vi "Drive Station HUD.vi"() -> ()   [LabVIEW 2018]
uses:
  <vilib>/Rock Robotics/Network Tables/NT Read Number.vi
  <vilib>/Rock Robotics/Network Tables/NT Read Boolean.vi
  <vilib>/vision/NI_Vision_Development_Module.lvlib
panel:
  out "Final Image":T1(plugin-control)
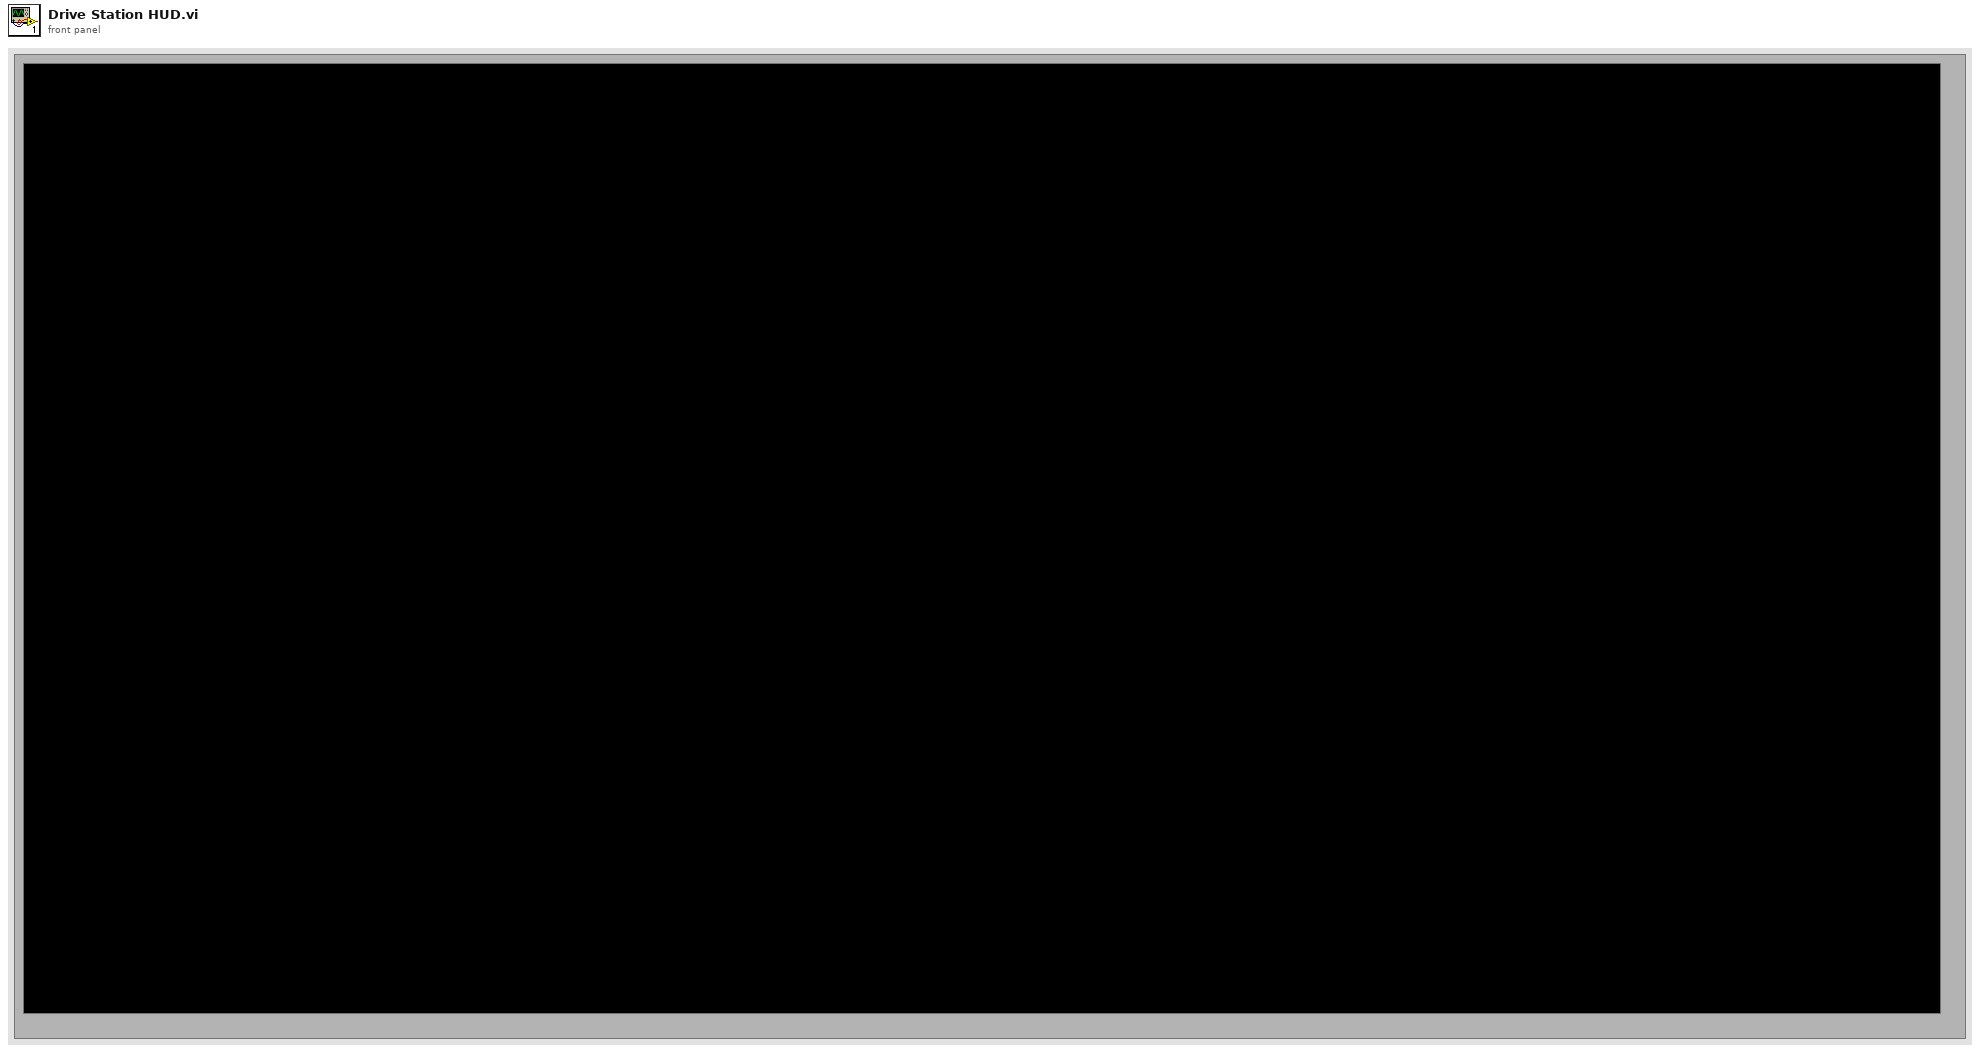
[diagram p1: front panel]
types:
  T1 = typedef "IMAQ Image.ctl" = refnum<image>
  T2 = enum32{"Invalid", "Standard", "Closed", "Hidden", "Minimized", "Maximized"}
  T3 = typedef "LVAllMonitorsDisplayTypeDef.ctl" = cluster{"Bounds":cluster{"Left":i16, "Top":i16, "Right":i16, "Bottom":i16}, "Depth":i16}[]
  T4 = cluster{"Left":i16, "Top":i16, "Right":i16, "Bottom":i16}
  T5 = cluster{"Left":i32, "Top":i32, "Right":i32, "Bottom":i32}
  T6 = cluster{"Desired Font (Application)":enum16{"User-specified Font", "Application Font", "System Font", "Dialog Font"}, "[User-specified Font]":cluster{"Font Name":string, "Size":i16, "Strikeout?":bool, "Italic?":bool, "Underline?":bool, "Outline?":bool, "Shadow?":bool, "Bold?":bool, "Rotation Angle":dbl}, "Horizontal Alignment":i16, "Vertical Alignment":i16}
  T7 = typedef "Image Type" = u32
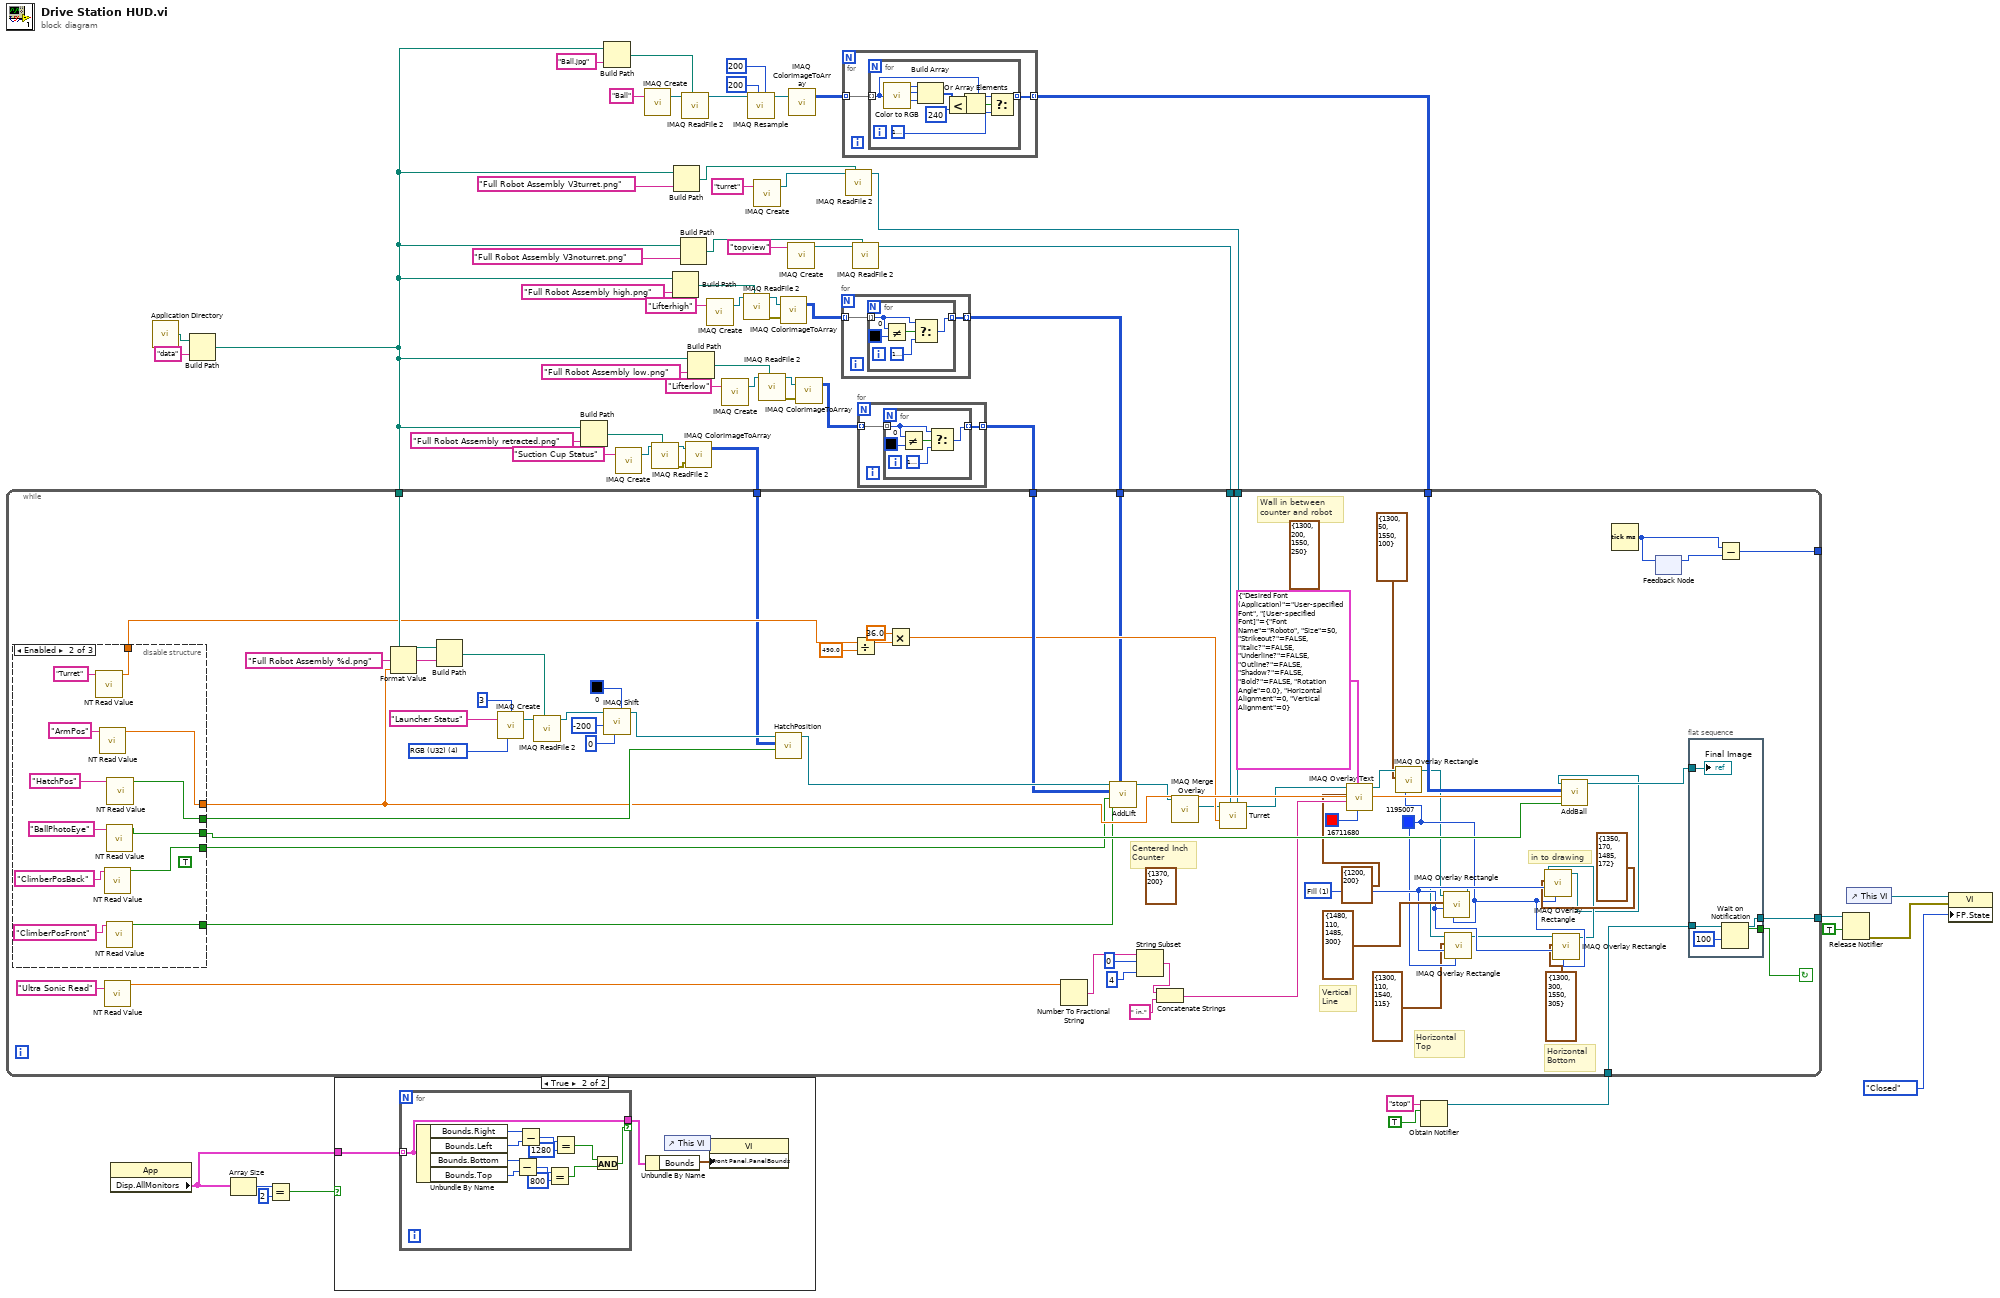
[diagram p0: block diagram]
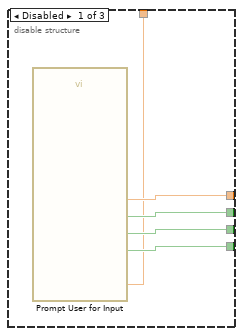
[diagram p2: hidden frame]
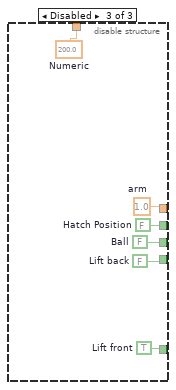
[diagram p3: hidden frame]
diagram:
  n1 = property class="App"() -> ("Disp.AllMonitors"=w55:T3)  [unwired: 2 in, 2 out]
  n2 = call <vilib>:"Application Directory.vi"() -> ("Application Directory"=w53:path)
  n3 = Build Path(base path=w53, name or relative path="data") -> (appended path=w1:path)
  n4 = Array Size(array=w55) -> (size(s)=w58:i32)
  n5 = Equal?(x=w58, y=2) -> (x = y?=w56:bool)
  n6 = case shown="True" w56 {
    tunnel: w55 -> [_ w62]
    frame False {
    }
    frame True {
      n7 = for {
        tunnel: w62 -> [w64] mode=indexing
        tunnel: [w64] -> w60 if=w63
        n8 = Unbundle By Name(w64) -> ("Bounds.Right"=w74:i16, "Bounds.Left"=w73:i16, "Bounds.Bottom"=w72:i16, "Bounds.Top"=w71:i16)
        n9 = Subtract(x=w72, y=w71) -> (x-y=w70:i16)
        n10 = Subtract(x=w74, y=w73) -> (x-y=w67:i16)
        n11 = Equal?(x=w70, y=i16 800) -> (x = y?=w65:bool)
        n12 = Equal?(x=w67, y=i16 1280) -> (x = y?=w66:bool)
        n13 = And(x=w66, y=w65) -> (x .and. y?=w63:bool)
      }
      n14 = Unbundle By Name(w60) -> ("Bounds"=w59:T4)
      n15 = control-ref of="This VI"() -> (w61:refnum<vi>)
      n16 = property class="VI"(reference=w61, "Front Panel.PanelBounds"=w59) -> ()  [unwired: 1 in, 2 out]
    }
  }
  n17 = Build Path(base path=w1, name or relative path="Full Robot Assembly retracted.png") -> (appended path=w14:path)
  n18 = Build Path(base path=w1, name or relative path="Ball.jpg") -> (appended path=w52:path)
  n19 = call "IMAQ Create"("Image Name"="Suction Cup Status") -> ("New Image"=w11:T1)  [unwired: 4 in, 1 out]
  n20 = call "IMAQ Create"("Image Name"="Ball") -> ("New Image"=w48:T1)  [unwired: 4 in, 1 out]
  n21 = call "IMAQ ReadFile 2"("File Path"=w14, "Image"=w11) -> ("error out"=w13:errorcluster, "Image Out"=w16:T1)  [unwired: 5 in, 3 out]
  n22 = Build Path(base path=w1, name or relative path="Full Robot Assembly high.png") -> (appended path=w2:path)
  n23 = Build Path(base path=w1, name or relative path="Full Robot Assembly V3turret.png") -> (appended path=w19:path)
  n24 = Build Path(base path=w1, name or relative path="Full Robot Assembly V3noturret.png") -> (appended path=w26:path)
  n25 = call "IMAQ ReadFile 2"("File Path"=w52, "Image"=w48) -> ("Image Out"=w49:T1)  [unwired: 5 in, 4 out]
  n26 = call "IMAQ ColorImageToArray"("Image"=w16, "error in (no error)"=w13) -> ("Image Pixels (U32)"=w10:u32[][])  [unwired: 2 in, 2 out]
  n27 = Build Path(base path=w1, name or relative path="Full Robot Assembly low.png") -> (appended path=w41:path)
  n28 = call "IMAQ Create"("Image Name"="Lifterhigh") -> ("New Image"=w5:T1)  [unwired: 4 in, 1 out]
  n29 = call "IMAQ Create"("Image Name"="Lifterlow") -> ("New Image"=w38:T1)  [unwired: 4 in, 1 out]
  n30 = call "IMAQ ReadFile 2"("File Path"=w2, "Image"=w5) -> ("error out"=w3:errorcluster, "Image Out"=w4:T1)  [unwired: 5 in, 3 out]
  n31 = call "IMAQ Resample"("X Resolution"=200, "Y Resolution"=200 ("X Resolution"), "Image Src"=w49) -> ("Image Dst Out"=w50:T1)  [unwired: 7 in, 1 out]
  n32 = call "IMAQ Create"("Image Name"="turret") -> ("New Image"=w20:T1)  [unwired: 4 in, 1 out]
  n33 = call "IMAQ ReadFile 2"("File Path"=w41, "Image"=w38) -> ("error out"=w40:errorcluster, "Image Out"=w39:T1)  [unwired: 5 in, 3 out]
  n34 = call "IMAQ ColorImageToArray"("Image"=w4, "error in (no error)"=w3) -> ("Image Pixels (U32)"=w9:u32[][])  [unwired: 2 in, 2 out]
  n35 = call "IMAQ Create"("Image Name"="topview") -> ("New Image"=w25:T1)  [unwired: 4 in, 1 out]
  n36 = call "IMAQ ColorImageToArray"("Image"=w50) -> ("Image Pixels (U32)"=w51:u32[][])  [unwired: 3 in, 2 out]
  n37 = call "IMAQ ColorImageToArray"("Image"=w39, "error in (no error)"=w40) -> ("Image Pixels (U32)"=w42:u32[][])  [unwired: 2 in, 2 out]
  n38 = for {
    tunnel: w9 -> [w76] mode=indexing
    tunnel: [w75] -> w8 mode=indexing
    n39 = for {
      tunnel: w76 -> [w79] mode=indexing
      tunnel: [w78] -> w75 mode=indexing
      n40 = Not Equal?(x=w79, y=u32 0) -> (x != y?=w80:bool)
      n41 = Select(t=w79, s=w80, f=u32 16777216) -> (s? t:f=w78:u32)
    }
  }
  n42 = for {
    tunnel: w51 -> [w83] mode=indexing
    tunnel: [w82] -> w43 mode=indexing
    n43 = for {
      tunnel: w83 -> [w85] mode=indexing
      tunnel: [w93] -> w82 mode=indexing
      n44 = call <vilib>:"Color to RGB.vi"("Color"=w85) -> ("Resolved Color"=w91:u32, "R"=w90:u8, "G"=w89:u8)  [unwired: 1 out]
      n45 = Build Array(w91, w90, w89) -> (w87:u32[])
      n46 = Less?(x=w87, y=240) -> (x < y?=w88:bool[])
      n47 = Or Array Elements(Boolean array=w88) -> (logical OR=w84:bool)
      n48 = Select(t=w85, s=w84, f=u32 16777216) -> (s? t:f=w93:u32)
    }
  }
  n49 = call "IMAQ ReadFile 2"("File Path"=w19, "Image"=w20) -> ("Image Out"=w17:T1)  [unwired: 5 in, 4 out]
  n50 = call "IMAQ ReadFile 2"("File Path"=w26, "Image"=w25) -> ("Image Out"=w22:T1)  [unwired: 5 in, 4 out]
  n51 = for {
    tunnel: w42 -> [w95] mode=indexing
    tunnel: [w94] -> w35 mode=indexing
    n52 = for {
      tunnel: w95 -> [w98] mode=indexing
      tunnel: [w97] -> w94 mode=indexing
      n53 = Not Equal?(x=w98, y=u32 0) -> (x != y?=w99:bool)
      n54 = Select(t=w98, s=w99, f=u32 16777216) -> (s? t:f=w97:u32)
    }
  }
  n55 = Obtain Notifier(name (unnamed)="stop", notification data type=TRUE) -> (notifier out=w32:refnum<notifier>)  [unwired: 2 in, 2 out]
  n56 = while {
    tunnel: w1 -> [w156]
    tunnel: w43 -> [w155]
    tunnel: w35 -> [w154]
    tunnel: w32 -> [w150]
    tunnel: [w149] -> w31
    tunnel: w22 -> [w134]
    tunnel: w17 -> [w132]
    tunnel: w10 -> [w130]
    tunnel: w8 -> [w129]
    tunnel: [w126] -> _
    stop <- w143 continue-if-true
    w110 = u32 1 items=["Frame", "Fill", "Highlight"] ("Drawing Mode (Frame)")
    (unwired) T5 {"Left"=1300, "Top"=200, "Right"=1550, "Bottom"=250} ("Rectangle")
    w107 = u32 1195007 ("Color")
    (unwired) cluster{"X":i32, "Y":i32} {"X"=1370, "Y"=200} ("Origin")
    w163 = T7 4 items=["Grayscale (U8)", "Grayscale (I16)", "Grayscale (SGL)", "Complex (CSG)", "RGB (U32)", "HSL (U32)", "RGB (U64)", "Grayscale (U16)"] ("Image Type")
    # "Horizontal\nBottom"
    # "Horizontal\nTop"
    # "Vertical\nLine"
    # "in to drawing"
    # "Centered Inch\nCounter"
    # "Wall in between \ncounter and robot"
    n57 = disable-structure shown="Enabled" {
      disable-tunnel: [w175 w183 w193] -> w153
      disable-tunnel: [w174 w184 w192] -> w152
      disable-tunnel: [w173 w186 w189] -> w151
      disable-tunnel: [w172 w185 w191] -> w142
      disable-tunnel: [w170 w177 w188] -> w148
      disable-tunnel: [_ w176 w190] -> w136
      frame Disabled {
        n58 = call "Prompt User for Input"() -> ("turret angle"=w170:dbl, "Invert Colors"=w171:bool, "Lifter extended"=w172:bool, "Ball Obtained"=w174:bool, "Suction Cup extended"=w175:bool, "Position of Launcher:"=w173:dbl)  [unwired: 12 in, 2 out]
      }
      frame Enabled {
        (unwired) TRUE ("Invert Colors")
        n59 = call-poly <vilib>:"NT Read Value.vi"("Name"="Turret") -> ("Numeric"=w177:dbl)  [unwired: 9 in, 1 out]
        n60 = call-poly <vilib>:"NT Read Value.vi"("Name"="ArmPos") -> ("Numeric"=w186:dbl)  [unwired: 9 in, 1 out]
        n61 = call-poly <vilib>:"NT Read Value.vi"("Name"="ClimberPosBack") -> ("Boolean"=w185:bool)  [unwired: 9 in, 1 out]
        n62 = call-poly <vilib>:"NT Read Value.vi"("Name"="BallPhotoEye") -> ("Boolean"=w184:bool)  [unwired: 9 in, 1 out]
        n63 = call-poly <vilib>:"NT Read Value.vi"("Name"="ClimberPosFront") -> ("Boolean"=w176:bool)  [unwired: 9 in, 1 out]
        n64 = call-poly <vilib>:"NT Read Value.vi"("Name"="HatchPos") -> ("Boolean"=w183:bool)  [unwired: 9 in, 1 out]
      }
      frame Disabled {
        w188 = 200.0  # Numeric
        w189 = 1.0  # arm
        w190 = TRUE  # Lift front
        w191 = FALSE  # Lift back
        w192 = FALSE  # Ball
        w193 = FALSE  # Hatch Position
      }
    }
    n65 = call-poly <vilib>:"NT Read Value.vi"("Name"="Ultra Sonic Read") -> ("Numeric"=w123:dbl)  [unwired: 9 in, 1 out]
    n66 = Format Value(format string="Full Robot Assembly %d.png", value (0)=w151) -> (output string=w159:string)  [unwired: 1 in]
    n67 = Build Path(base path=w156, name or relative path=w159) -> (appended path=w158:path)
    n68 = call "IMAQ Create"("Border Size"=3, "Image Name"="Launcher Status", "Image Type"=w163) -> ("New Image"=w162:T1)  [unwired: 2 in, 1 out]
    n69 = call "IMAQ ReadFile 2"("File Path"=w158, "Image"=w162) -> ("Image Out"=w140:T1)  [unwired: 5 in, 4 out]
    n70 = call "IMAQ Shift"("Color Replace Value"=u32 0, "YOffset"=0, "XOffset"=-200, "Image Src"=w140) -> ("Image Dst Out"=w141:T1)  [unwired: 6 in, 1 out]
    n71 = call "HatchPosition.vi"("Boolean"=w153, "Bitmap"=w130, "Refnum in"=w141) -> ("Refnum out"=w157:T1)  [unwired: 8 in]
    n72 = Divide(x=w148, y=490.0) -> (x/y=w147:dbl)
    n73 = Multiply(x=36.0, y=w147) -> (x*y=w131:dbl)
    n74 = Number To Fractional String(number=w123) -> (F-format string=w118:string)  [unwired: 3 in]
    n75 = call "AddLift.vi"("ArrayHigh"=w129, "Front"=w136, "Back"=w142, "ArrayLow"=w154, "Refnum in"=w157) -> ("Refnum out"=w133:T1)  [unwired: 6 in]
    n76 = String Subset(string=w118, offset (0)=0, length (rest)=4 ("length (rest)")) -> (substring=w115:string)
    n77 = Concatenate Strings(w115, " in." ("string")) -> (w119:string)
    n78 = call "IMAQ Merge Overlay"("Image Src"=w133) -> ("Image Dst Out"=w125:T1)  [unwired: 9 in, 1 out]
    n79 = call "Turret.vi"("turret"=w132, "top view"=w134, "angle"=w131, "Refnum in"=w125) -> ("Refnum out"=w135:T1)  [unwired: 7 in]
    n80 = call "IMAQ Overlay Text"("Text Color (black)"=u32 16711680, "Font, Size & Style"=T6 {"Desired Font (Application)"=enum."User-specified Font", "[User-specified Font]"={"Font Name"="Roboto", "Size"=50, "Strikeout?"=FALSE, "Italic?"=FALSE, "Underline?"=FALSE, "Outline?"=FALSE, "Shadow?"=FALSE, "Bold?"=FALSE, "Rotation Angle"=0.0}, "Horizontal Alignment"=0, "Vertical Alignment"=0}, "String"=w119, "Origin"=cluster{"X":i32, "Y":i32} {"X"=1200, "Y"=200}, "Image"=w135) -> ("Image Out"=w114:T1)  [unwired: 5 in, 1 out]
    n81 = call "IMAQ Overlay Rectangle"("Color"=w107, "Rectangle"=T5 {"Left"=1300, "Top"=50, "Right"=1550, "Bottom"=100}, "Image"=w114) -> ("Image Out"=w106:T1)  [unwired: 7 in, 1 out]
    n82 = call "IMAQ Overlay Rectangle"("Color"=w107, "Drawing Mode (Frame)"=w110, "Rectangle"=T5 {"Left"=1480, "Top"=110, "Right"=1485, "Bottom"=300}, "Image"=w106) -> ("Image Out"=w105:T1)  [unwired: 6 in, 1 out]
    n83 = call "IMAQ Overlay Rectangle"("Color"=w107, "Drawing Mode (Frame)"=w110, "Rectangle"=T5 {"Left"=1300, "Top"=110, "Right"=1540, "Bottom"=115}, "Image"=w105) -> ("Image Out"=w104:T1)  [unwired: 6 in, 1 out]
    n84 = call "IMAQ Overlay Rectangle"("Color"=w107, "Drawing Mode (Frame)"=w110, "Rectangle"=T5 {"Left"=1300, "Top"=300, "Right"=1550, "Bottom"=305}, "Image"=w104) -> ("Image Out"=w103:T1)  [unwired: 6 in, 1 out]
    n85 = call "IMAQ Overlay Rectangle"("Color"=w107, "Drawing Mode (Frame)"=w110, "Rectangle"=T5 {"Left"=1350, "Top"=170, "Right"=1485, "Bottom"=172}, "Image"=w103) -> ("Image Out"=w102:T1)  [unwired: 6 in, 1 out]
    n86 = call "AddBall.vi"("Boolean"=w152, "Numeric"=w151, "Array"=w155, "Refnum in"=w102) -> ("Refnum out"=w144:T1)  [unwired: 7 in]
    n87 = Tick Count (ms)() -> (millisecond timer value=w128:u32)
    n88 = feedback-in #1(w128) -> ()
    n89 = feedback #1() -> (w127:u32)  [unwired: 1 in]
    n90 = flat-sequence {
      tunnel: [w169] -> w143
      tunnel: w150 -> [w168]
      tunnel: [w166] -> w149
      tunnel: w144 -> [w165]
      frame #0 {
        n91 = Wait on Notification(notifier=w168, timeout in ms (-1)=100) -> (notifier out=w166:refnum<notifier>, timed out?=w169:bool)  [unwired: 2 in, 2 out]
        "Final Image" <- w165
      }
    }
    n92 = Subtract(x=w128, y=w127) -> (x-y=w126:u32)
  }
  n93 = Release Notifier(notifier=w31, force destroy? (F)=TRUE) -> (error out=w27:errorcluster)  [unwired: 1 in, 2 out]
  n94 = control-ref of="This VI"() -> (w29:refnum<vi>)
  n95 = property class="VI"(reference=w29, error in=w27, "FP.State"=T2."Closed" ("Front Panel Window:State")) -> ()  [unwired: 2 out]
